vi "RSZVB Get Fundamental Frequency Signal.vi"(8 "error in (no error)":errorcluster {"code" format="%.0x"}, 10 "Channel (1)":i32=1, 11 "VISA session":refnum<visa-resource-name>) -> (0 "error out":errorcluster {"code" format="%.0x"}, 2 "Fundamental Frequency":i32, 3 "dup VISA session":refnum<visa-resource-name>)   [LabVIEW 2011]
doc: "This VI returns the mixer input or output signal which is at the fundamental frequency .\n\nRemote-control command(s):\n[SENSe<Ch>:]FREQuency:CONVersion:MIXer:FUNDamental?"
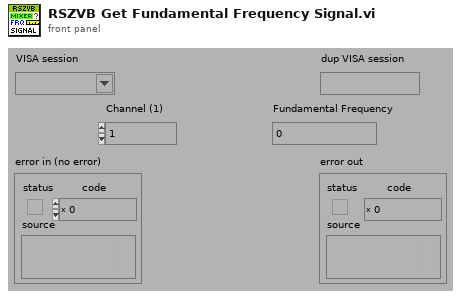
[diagram p1: front panel]
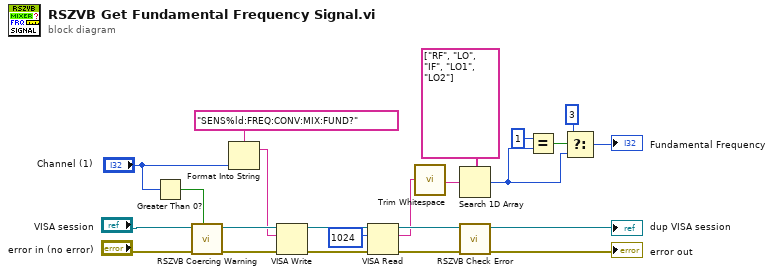
[diagram p0: block diagram]
diagram:
  n1 = Greater Than 0?(x="Channel (1)") -> (x > 0?=w14:bool)
  n2 = call "RSZVB Coercing Warning.vi"("In Range?"=w14, "error in (no error)"="error in (no error)", "VISA session"="VISA session") -> ("error out"=w21:errorcluster, "dup VISA session"=w22:refnum<visa-resource-name>)  [unwired: 7 in]
  n3 = Format Into String(format string="SENS%ld:FREQ:CONV:MIX:FUND?", "Channel (1)") -> (resulting string=w20:string)  [unwired: 2 in, 1 out]
  n4 = VISA Write(VISA resource name=w22, write buffer=w20, error in (no error)=w21) -> (VISA resource name out=w17:refnum<visa-resource-name>, error out=w19:errorcluster)  [unwired: 1 out]
  n5 = VISA Read(VISA resource name=w17, byte count=u32 1024 ("byte count (0)"), error in (no error)=w19) -> (VISA resource name out=w16:refnum<visa-resource-name>, read buffer=w11:string, error out=w15:errorcluster)  [unwired: 1 out]
  n6 = call <vilib>:"Trim Whitespace.vi"("string"=w11) -> ("trimmed string"=w12:string)  [unwired: 1 in]
  n7 = Search 1D Array(1D array=string[] ["RF", "LO", "IF", "LO1", "LO2"] ("array 2"), element=w12) -> (index of element=w3:i32)  [unwired: 1 in]
  n8 = call "RSZVB Check Error.vi"("error in (no error)"=w15, "VISA session"=w16) -> ("error out"=→"error out":errorcluster, "dup VISA session"=→"dup VISA session":refnum<visa-resource-name>)  [unwired: 8 in]
  n9 = Equal?(x=1, y=w3) -> (x = y?=w4:bool)
  n10 = Select(t=3, s=w4, f=w3) -> (s? t:f=→"Fundamental Frequency":i32)
